vi "Raise stop flag.vi"(8 "error in (no error)":errorcluster, 10 "on/off":bool, 11 "Monkey in":refnum<class "Monkey.lvclass">) -> (0 "error out":errorcluster, 3 "Monkey out":refnum<class "Monkey.lvclass">)   [LabVIEW 2020, in "TALOS.lvlib" / "Monkey.lvlib" / "Monkey.lvclass"]
doc: "Set the stop flag and show/hide indicators"
uses:
  Monkey.lvclass
  C:/LabVIEW Code/TALOS/talos/Father of all uServices/Father of all uServices/Father of all uServices.lvclass
  Monkey.lvclass/Monkey.ctl
  Father of all uServices/Father of all uServices/Father of all uServices.lvclass
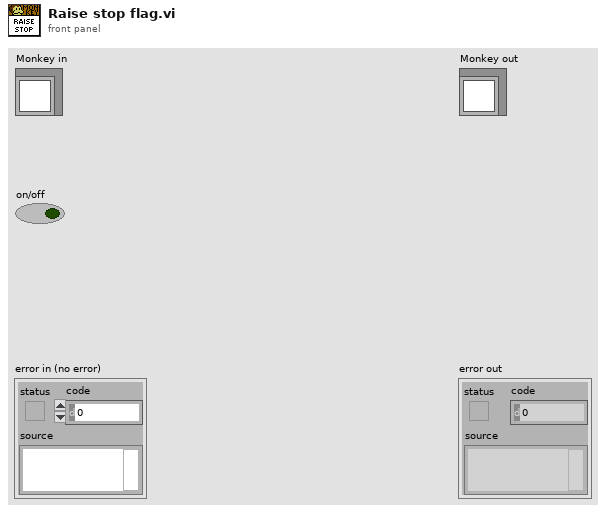
[diagram p1: front panel]
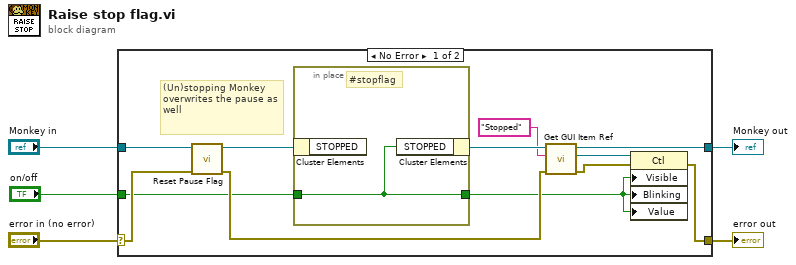
[diagram p0: block diagram]
diagram:
  n1 = case shown="No Error" "error in (no error)" {
    selector: "error in (no error)" -> [w16 w20]
    tunnel: [w8 w20] -> w4
    tunnel: [w9 w19] -> w2
    tunnel: "Monkey in" -> [w7 w19]
    tunnel: "on/off" -> [w11 _]
    frame No Error {
      # "(Un)stopping Monkey overwrites the pause as well"
      n2 = call-dynamic "Reset Pause Flag.vi"("error in (no error)"=w16, "Monkey in"=w7) -> ("error out"=w17:errorcluster, "Monkey out"=w6:refnum<class "Monkey.lvclass">)  [unwired: 8 in]
      n3 = in-place {
        in-place-border: w11 -> [w18]
        in-place-border: [w18] -> w10
        # "#stopflag"
        n4 = in-place-cluster #1(w6) -> ()  [unwired: 1 out]
        n5 = in-place-cluster #1("STOPPED"=w18) -> (w13:refnum<class "Monkey.lvclass">)
      }
      n6 = call "Get GUI Item Ref.vi"("error in (no error)"=w17, "FP Item Name"="Stopped", "uService Template in"=w13) -> ("error out"=w14:errorcluster, "Ctl Refnum"=w15:refnum<vi>, "uService Template out"=w9:refnum<class "Monkey.lvclass">)  [unwired: 6 in]
      n7 = property class="Ctl"(reference=w15, error in=w14, "Visible"=w10, "Blinking"=w10, "Value"=w10) -> (error out=w8:errorcluster)  [unwired: 1 out]
    }
    frame Error {
    }
  }
  "error out" <- w4
  "Monkey out" <- w2
